vi "getItem.vi"(8 "error in (no error)":errorcluster, 10 "Key":string, 11 "HashMap in":refnum<class "HashMap.lvclass">) -> (0 "error out":errorcluster, 2 "Value":variant, 3 "HashMap out":refnum<class "HashMap.lvclass">)   [LabVIEW 2017, in "HashMap.lvclass"]
uses:
  <userlib>/836-Library/Data_Structures/HashMap/HashMap.lvclass
  <userlib>/836-Library/Data_Structures/HashMap/HashMap.lvclass/HashMap.ctl
  <vilib>/ErrorRing/Error Ring.xnode
  <userlib>/836-Library/Data_Structures/Bucket/Bucket.lvclass
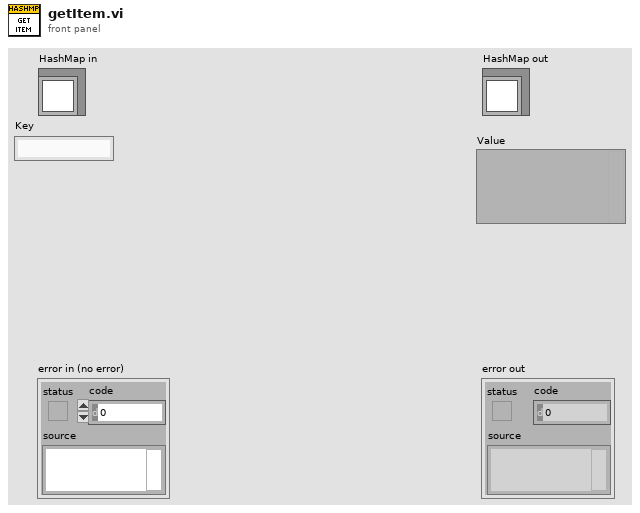
[diagram p1: front panel]
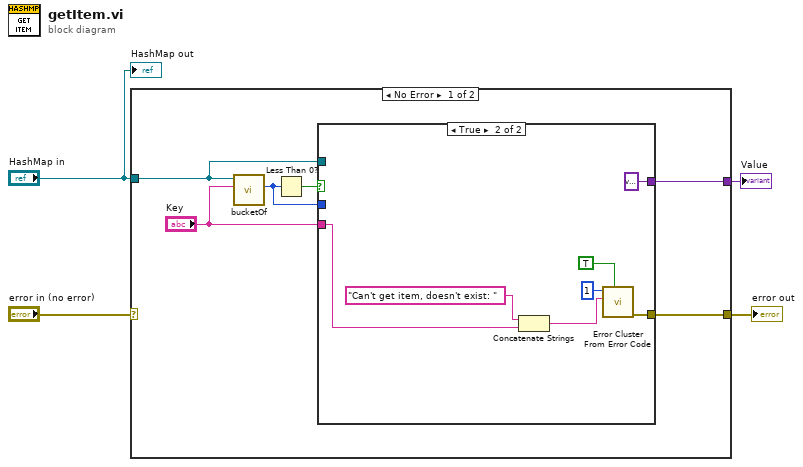
[diagram p0: block diagram]
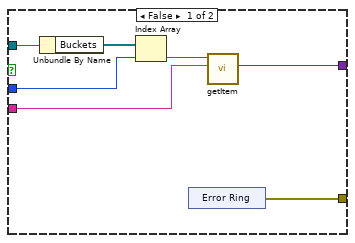
[diagram p2: hidden frame]
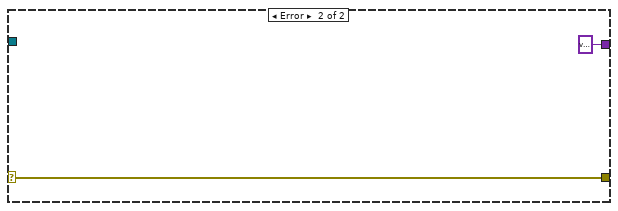
[diagram p3: hidden frame]
diagram:
  n1 = case shown="No Error" "error in (no error)" {
    selector: "error in (no error)" -> [_ w27]
    tunnel: [w5 w27] -> w3
    tunnel: "HashMap in" -> [w8 _]
    tunnel: [w6 variant ("Value")] -> w1
    frame No Error {
      n2 = call <userlib>:"bucketOf.vi"("Key"="Key", "HashMap in"=w8) -> ("Bucket Index"=w9:i32)  [unwired: 7 in, 2 out]
      n3 = Less Than 0?(x=w9) -> (x < 0?=w10:bool)
      n4 = case shown="True" w10 {
        tunnel: w9 -> [w15 _]
        tunnel: w8 -> [w17 _]
        tunnel: "Key" -> [w12 w20]
        tunnel: [w13 variant ("Value")] -> w6
        tunnel: [w11 w24] -> w5
        frame False {
          n5 = Unbundle By Name(w17) -> ("Buckets"=w16:refnum<class "Bucket.lvclass">[])
          n6 = Index Array(array=w16, index=w15) -> (element=w14:refnum<class "Bucket.lvclass">)
          n7 = xnode "Error Ring"() -> ("error out"=w11:errorcluster)
          n8 = call <userlib>:"getItem.vi"("Key"=w12, "Bucket in"=w14) -> ("Value"=w13:variant)  [unwired: 7 in, 2 out]
        }
        frame True {
          n9 = Concatenate Strings("Can't get item, doesn't exist: " ("string"), w20) -> (w21:string)
          n10 = call <vilib>:"Error Cluster From Error Code.vi"("show call chain? (False)"=TRUE, "error message (\"\")"=w21, "error code (0)"=1) -> ("error out"=w24:errorcluster)  [unwired: 6 in]
        }
      }
    }
    frame Error {
    }
  }
  "error out" <- w3
  "Value" <- w1
  "HashMap out" <- "HashMap in"
